vi "HRTF-Launcher.vi"() -> ()   [LabVIEW 2015]
uses:
  <resource>/objmgr/daqmx.rc
panel:
  out "Loading":string
  out "Version":string
  # "HRTF Measurement"
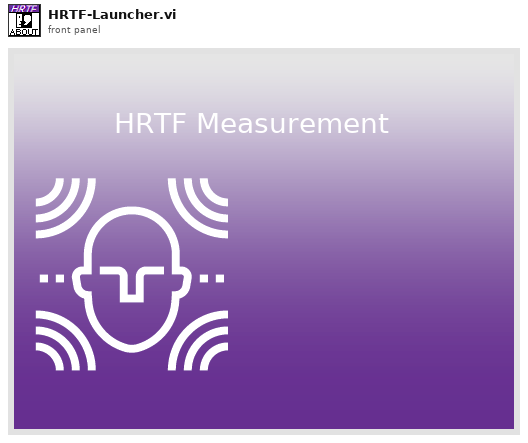
[diagram p1: front panel]
types:
  T1 = cluster{"Major":i32, "Minor":i32, "Build":i32, "Private":i32, "FileVersion":string, "ProductName":string, "InternalName":string, "CompanyName":string, "LegalCopyright":string, "FileDescription":string}
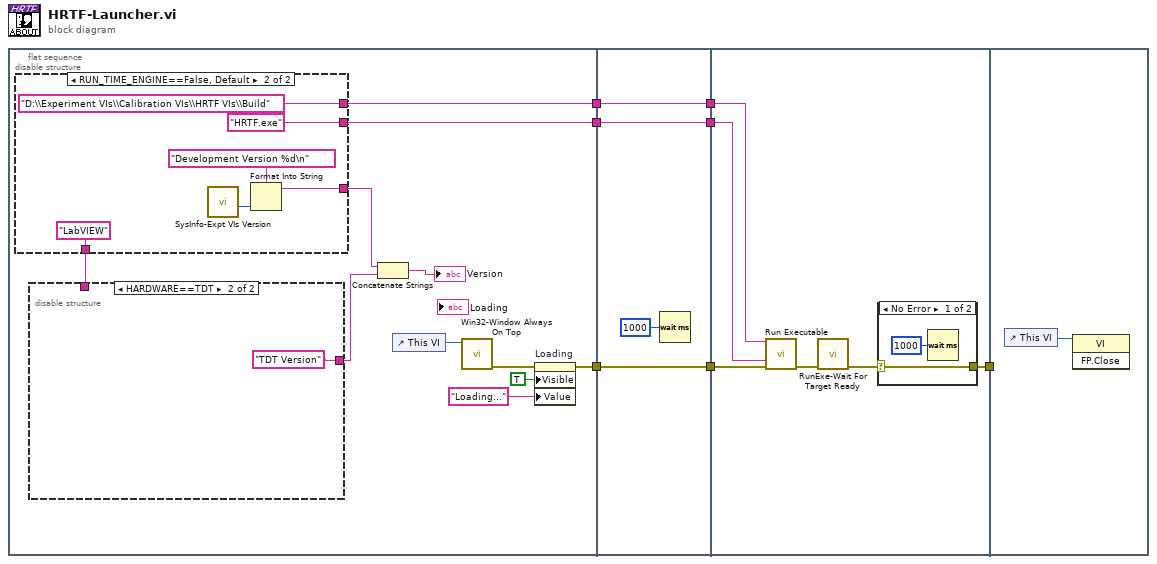
[diagram p0: block diagram]
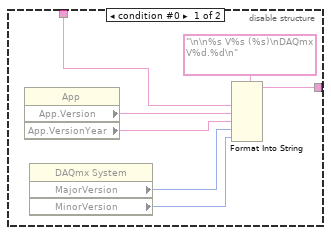
[diagram p2: hidden frame]
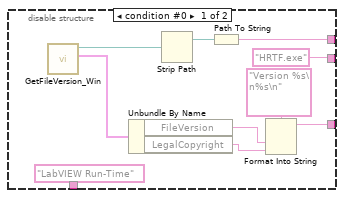
[diagram p3: hidden frame]
diagram:
  n1 = flat-sequence {
    tunnel: [w16] -> w7
    tunnel: [w14] -> w6
    tunnel: [w13] -> w5
    tunnel: [w46] -> w4
    tunnel: w7 -> [w46]
    tunnel: [w45] -> w3
    tunnel: w6 -> [w45]
    tunnel: [w44] -> w2
    tunnel: w5 -> [w44]
    tunnel: w4 -> [w50]
    tunnel: w3 -> [w49]
    tunnel: w2 -> [w48]
    tunnel: [w47] -> w1
    tunnel: w1 -> [_]
    frame #0 {
      n2 = disable-structure shown="RUN_TIME_ENGINE==False, Default" {
        disable-tunnel: [w34 w40] -> w12
        disable-tunnel: ["LabVIEW Run-Time" "LabVIEW"] -> w8
        disable-tunnel: [w27 "D:\\Experiment VIs\\Calibration VIs\\HRTF VIs\\Build" ("Folder")] -> w14
        disable-tunnel: ["HRTF.exe" (".EXE name") "HRTF.exe" (".EXE name")] -> w13
        frame condition #0 {
          n3 = call "GetFileVersion_Win.vi"() -> ("File Info Out"=w35:T1, "Exe Path Out"=w30:path)  [unwired: 9 in, 1 out]
          n4 = Unbundle By Name(w35) -> ("FileVersion"=w33:string, "LegalCopyright"=w32:string)
          n5 = Strip Path(path=w30) -> (stripped path=w28:path)  [unwired: 1 out]
          n6 = Path To String(path=w28) -> (string=w27:string)
          n7 = Format Into String(format string="Version %s\n%s\n", w33, w32) -> (resulting string=w34:string)  [unwired: 2 in, 1 out]
        }
        frame condition #1 (active) {
          n8 = call "SysInfo-Expt VIs Version.vi"() -> ("Expt VIs Version out"=w41:i32)  [unwired: 11 in]
          n9 = Format Into String(format string="Development Version %d\n" ("PF Version"), w41) -> (resulting string=w40:string)  [unwired: 2 in, 1 out]
        }
      }
      n10 = disable-structure shown="HARDWARE==TDT" {
        disable-tunnel: [w21 "TDT Version"] -> w9
        disable-tunnel: w8 -> [w22 _]
        frame condition #0 {
          n11 = property class="App"() -> ("App.Version"=w24:string, "App.VersionYear"=w23:string)  [unwired: 2 in, 2 out]
          n12 = property class="DAQmx System"() -> ("MajorVersion"=w20:u32, "MinorVersion"=w19:u32)  [unwired: 2 in, 2 out]
          n13 = Format Into String(format string="\n\n%s V%s (%s)\nDAQmx V%d.%d\n", w22, w24, w23, w20, w19) -> (resulting string=w21:string)  [unwired: 2 in, 1 out]
        }
        frame condition #1 (active) {
        }
      }
      n14 = Concatenate Strings(w12, w9) -> (→"Version":string)
      n15 = control-ref of="This VI"() -> (w11:refnum<vi>)
      n16 = call "Win32-Window Always On Top.vi"("VI reference"=w11) -> ("error out"=w15:errorcluster)  [unwired: 10 in]
      n17 = property on="Loading" class="Str"(error in=w15, "Visible"=TRUE, "Value"="Loading..." ("Loading")) -> (error out=w16:errorcluster)  [unwired: 1 in, 1 out]
    }
    frame #1 {
      n18 = Wait (ms)(milliseconds to wait=u32 1000) -> ()  [unwired: 1 out]
    }
    frame #2 {
      n19 = call "Run Executable.vi"("Folder"=w49, ".EXE name"=w48, "error in (no error)"=w50) -> ("error out"=w51:errorcluster)  [unwired: 12 in]
      n20 = call "RunExe-Wait For Target Ready.vi"("error in (no error)"=w51) -> ("error out"=w52:errorcluster)  [unwired: 14 in]
      n21 = case shown="No Error" w52 {
        selector: w52 -> [w53 w55]
        tunnel: [w53 w55] -> w47
        frame No Error {
          n22 = Wait (ms)(milliseconds to wait=u32 1000) -> ()  [unwired: 1 out]
        }
        frame Error {
        }
      }
    }
    frame #3 {
      n23 = control-ref of="This VI"() -> (w56:refnum<vi>)
      n24 = invoke class="VI" method="FP.Close"(reference=w56) -> ()  [unwired: 2 in, 3 out]
    }
  }
